vi "Convert Channel Values to Static Generate Digital Settings.vi"(9 "Length":i32, 10 "Index":i32, 11 "Channel Values in":dbl[](array[numeric])) -> (2 "Static Generate Digital Settings":T1, 3 "Channel Values out":dbl[](array[numeric]))   [LabVIEW 2018, in "FPGA Addon Engine.lvlib"]
uses:
  FPGA Addon Engine.lvlib
  Submodules/Source/Types/Static.Generate.Digital.Settings.ctl
  Submodules/Source/Speciality FPGA IO.lvlib
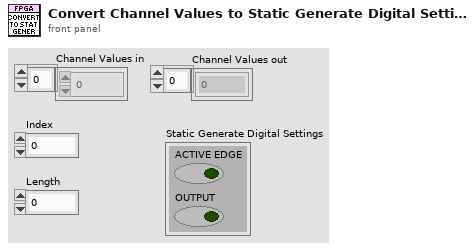
[diagram p1: front panel]
types:
  T1 = typedef "Speciality FPGA IO.lvlib/Static.Generate.Digital.Settings.ctl" = cluster{"ACTIVE EDGE":bool, "OUTPUT":bool}
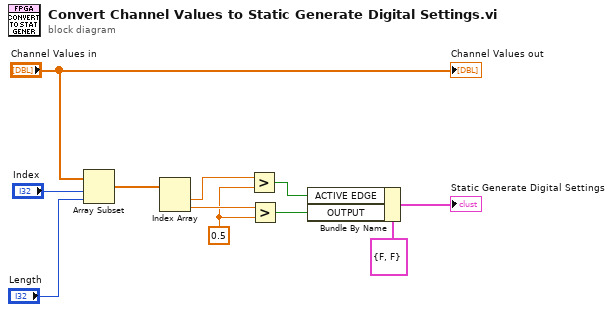
[diagram p0: block diagram]
diagram:
  w3 = 0.5 ("y")
  n1 = Array Subset(array="Channel Values in", index="Index", length="Length") -> (w1:dbl[])
  n2 = Index Array(array=w1) -> (element #1=w2:dbl, element #2=w4:dbl)  [unwired: 2 in]
  n3 = Greater?(x=w2, y=w3) -> (0:w5:bool)
  n4 = Greater?(x=w4, y=w3) -> (0:w11:bool)
  n5 = Bundle By Name(cluster=T1 {"ACTIVE EDGE"=FALSE, "OUTPUT"=FALSE} ("Settings"), "ACTIVE EDGE"=w5, "OUTPUT"=w11) -> (→"Static Generate Digital Settings":T1)
  "Channel Values out" <- "Channel Values in"
